vi "SeCrTs-AI Continuous Sequence Check.vi"(9 "output cluster":T1, 10 "AI":dbl, 11 "CDT":dbl) -> (1 "Failure case Seq":string, 2 "Boolean Range":bool, 3 "In Range":string)   [LabVIEW 2022 SP3]
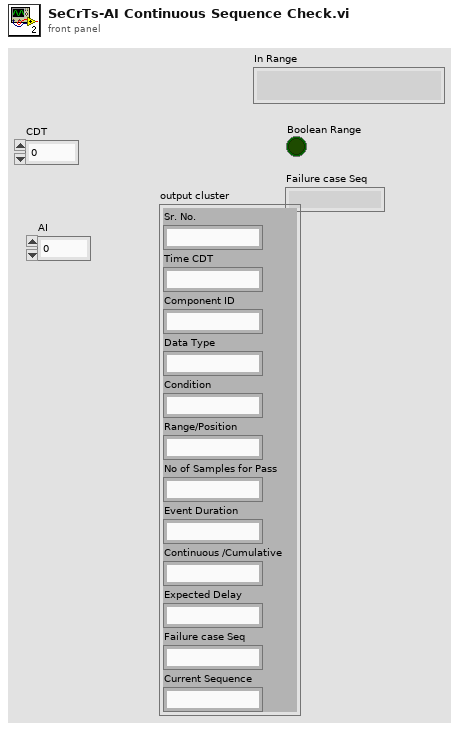
[diagram p1: front panel]
types:
  T1 = cluster{"Sr. No.":string, "Time CDT":string, "Component ID":string, "Data Type":string, "Condition":string, "Range/Position":string, "No of Samples for Pass":string, "Event Duration":string, "Continuous /Cumulative":string, "Expected Delay":string, "Failure case Seq":string, "Current Sequence":string}
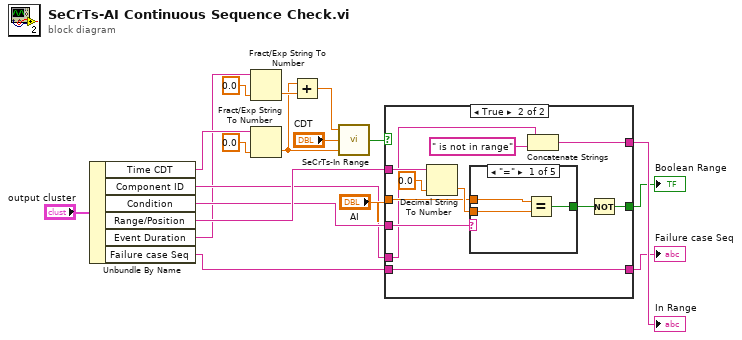
[diagram p0: block diagram]
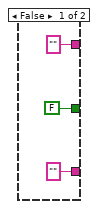
[diagram p2: hidden frame]
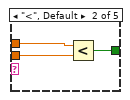
[diagram p3: hidden frame]
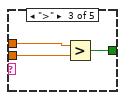
[diagram p4: hidden frame]
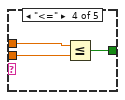
[diagram p5: hidden frame]
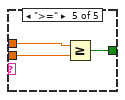
[diagram p6: hidden frame]
diagram:
  n1 = Unbundle By Name("output cluster") -> ("Time CDT"=w9:string, "Component ID"=w11:string, "Condition"=w12:string, "Range/Position"=w13:string, "Event Duration"=w5:string, "Failure case Seq"=w8:string)
  n2 = Fract/Exp String To Number(string=w5, default (0 dbl)=0.0) -> (number=w4:dbl)  [unwired: 2 in, 1 out]
  n3 = Fract/Exp String To Number(string=w9, default (0 dbl)=0.0) -> (number=w1:dbl)  [unwired: 2 in, 1 out]
  n4 = Add(x=w1, y=w4) -> (x+y=w3:dbl)
  n5 = call "SeCrTs-In Range.vi"("Min"=w1, "X"="CDT", "Max"=w3) -> ("In Range"=w7:bool)  [unwired: 2 in]
  n6 = case shown="True" w7 {
    tunnel: w13 -> [_ w32]
    tunnel: w12 -> [_ w30]
    tunnel: "AI" -> [_ w28]
    tunnel: w11 -> [_ w26]
    tunnel: ["" w25] -> w18
    tunnel: [FALSE w23] -> w17
    tunnel: w8 -> [_ w22]
    tunnel: ["" ("Failure case Seq") w22] -> w16
    frame False {
    }
    frame True {
      n7 = Decimal String To Number(string=w32, default (0L)=0.0) -> (number=w29:dbl)  [unwired: 1 in, 1 out]
      n8 = case shown="\"=\"" w30 {
        tunnel: w29 -> [w35 w37 w40 w43 w46]
        tunnel: w28 -> [w34 w38 w41 w44 w47]
        tunnel: [w33 w36 w39 w42 w45] -> w24
        frame "=" {
          n9 = Equal?(x=w34, y=w35) -> (x = y?=w33:bool)
        }
        frame "<", Default {
          n10 = Less?(x=w38, y=w37) -> (x < y?=w36:bool)
        }
        frame ">" {
          n11 = Greater?(x=w41, y=w40) -> (0:w39:bool)
        }
        frame "<=" {
          n12 = Less Or Equal?(x=w44, y=w43) -> (x <= y?=w42:bool)
        }
        frame ">=" {
          n13 = Greater Or Equal?(x=w47, y=w46) -> (x >= y?=w45:bool)
        }
      }
      n14 = Concatenate Strings(w26, " is not in range" ("string")) -> (w25:string)
      n15 = Not(x=w24) -> (.not. x?=w23:bool)
    }
  }
  "In Range" <- w18
  "Boolean Range" <- w17
  "Failure case Seq" <- w16
